vi "get index definition.vi"(10 "channel classification":T1, 11 "fixed channel configuration in":refnum<class "Watchdog configuration.lvclass">) -> (1 "valid?":bool, 2 "index cluster":variant, 3 "fixed channel configuration out":refnum<class "Watchdog configuration.lvclass">)   [LabVIEW 2013, in "Watchdog configuration.lvclass"]
uses:
  Watchdog configuration.lvclass
  <vilib>/NI/Tag Bus Module Framework/channel/channel classification.ctl
  <vilib>/NI/DCAF/Tag Editor Core/control module/configuration/control module configuration.lvclass
  <vilib>/NI/Tag Bus Module Framework/channel/TBM channel.lvclass
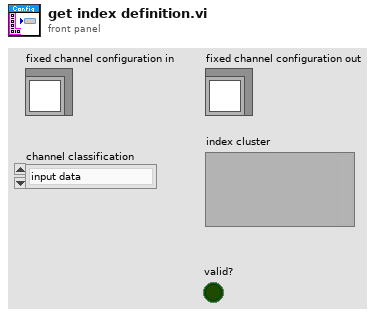
[diagram p1: front panel]
types:
  T1 = typedef "TBM channel.lvclass/channel classification.ctl" = enum16{"input data", "output data", "processing parameter", "processing result"}
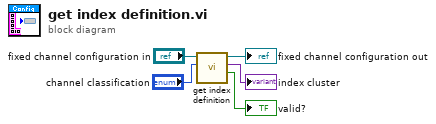
[diagram p0: block diagram]
diagram:
  n1 = call-parent "get index definition.vi"("channel classification"="channel classification", "fixed channel configuration in"="fixed channel configuration in") -> ("valid?"=→"valid?":bool, "index cluster"=→"index cluster":variant, "fixed channel configuration out"=→"fixed channel configuration out":refnum<class "Watchdog configuration.lvclass">)  [unwired: 7 in]
